vi "lab session 3.3.vi"() -> ()   [LabVIEW 2020]
panel:
  out "NOT(X2) OR NOT(Y2)":bool
  out "NOT(X2 AND Y2)":bool
  in  "Y 2":bool
  in  "X 2":bool
  out "NOT(X1) AND NOT(Y1)":bool
  out "NOT(X1 OR Y1)":bool
  in  "Y1":bool
  in  "X1":bool
  # "NOT(X.Y)=NOT(X)+NOT(Y)"
  # "NOT(X+Y)=NOT(X).NOT(Y)"
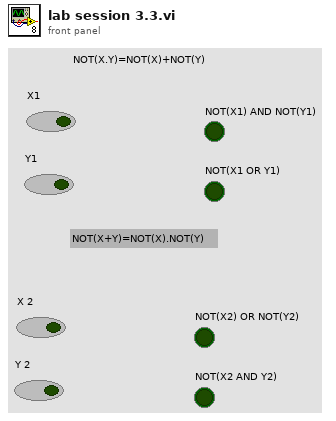
[diagram p1: front panel]
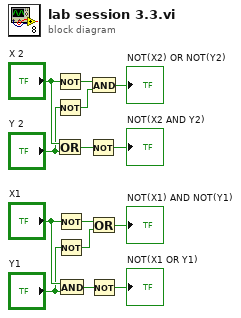
[diagram p0: block diagram]
diagram:
  n1 = Not(x="X 2") -> (.not. x?=w5:bool)
  n2 = Not(x="Y 2") -> (.not. x?=w4:bool)
  n3 = Or(x="X 2", y="Y 2") -> (x .or. y?=w1:bool)
  n4 = Not(x="X1") -> (.not. x?=w10:bool)
  n5 = Not(x="Y1") -> (.not. x?=w9:bool)
  n6 = And(x="X1", y="Y1") -> (x .and. y?=w14:bool)
  n7 = Not(x=w1) -> (.not. x?=→"NOT(X2 AND Y2)":bool)
  n8 = And(x=w5, y=w4) -> (x .and. y?=→"NOT(X2) OR NOT(Y2)":bool)
  n9 = Or(x=w10, y=w9) -> (x .or. y?=→"NOT(X1) AND NOT(Y1)":bool)
  n10 = Not(x=w14) -> (.not. x?=→"NOT(X1 OR Y1)":bool)
